vi "Convert Sensor Values.vi"(11 "ECE Units":dbl[](array[numeric])) -> (3 "CBME Units":dbl[](array[numeric]))   [LabVIEW 2016]
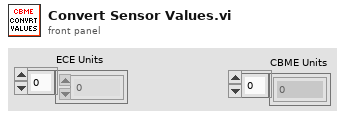
[diagram p1: front panel]
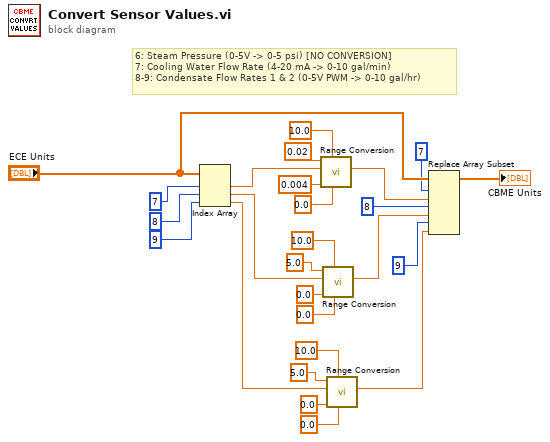
[diagram p0: block diagram]
diagram:
  # "6: Steam Pressure (0-5V -> 0-5 psi) [NO CONVERSION]\n7: Cooling Water Flow Rate (4-20 mA -> 0-10 gal/min)\n8-9: Condensate Flow Rates 1 & 2 (0-5V PWM -> 0-10 gal/hr)"
  n1 = Index Array(array="ECE Units", index #1=7 ("index"), index #2=8 ("index"), index #3=9 ("index")) -> (element #1=w23:dbl, element #2=w18:dbl, element #3=w9:dbl)
  n2 = call "Range Conversion.vi"("New Min"=0.0, "New Max"=10.0, "Current Min"=0.004, "Input Value"=w23, "Current Max"=0.02) -> ("Scaled Output"=w6:dbl)  [unwired: 6 in]
  n3 = call "Range Conversion.vi"("New Min"=0.0, "New Max"=10.0, "Current Min"=0.0, "Input Value"=w18, "Current Max"=5.0) -> ("Scaled Output"=w2:dbl)  [unwired: 6 in]
  n4 = call "Range Conversion.vi"("New Min"=0.0, "New Max"=10.0, "Current Min"=0.0, "Input Value"=w9, "Current Max"=5.0) -> ("Scaled Output"=w3:dbl)  [unwired: 6 in]
  n5 = Replace Array Subset(array="ECE Units", new element #1=w6, index #1=7 ("index"), new element #2=w2, index #2=8 ("index"), new element #3=w3, index #3=9 ("index")) -> (→"CBME Units":dbl[])
